vi "flatten parameters.vi"(8 "Output Tag":string, 9 "Process Variable Tag":string, 10 "Setpoint Tag":string, 11 "ID":string) -> (3 "wrapped data":string)   [LabVIEW 2014, in "PID Loop.lvclass"]
uses:
  PID Loop.lvclass
  String Parameters.ctl
  <vilib>/NI/Configuration Framework/serializable configuration/NISE_CEF_serializable configuration.lvclass
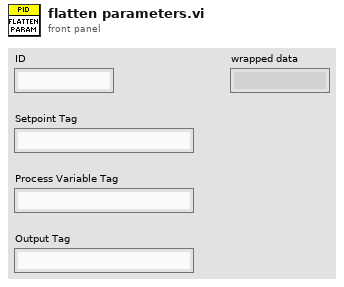
[diagram p1: front panel]
types:
  T1 = typedef "PID Loop.lvclass/String Parameters.ctl" = enum16{"Setpoint", "Process Variable", "Output", "Proportional Gain", "Integral Time", "Derivative Time", "Range High", "Range Low"}
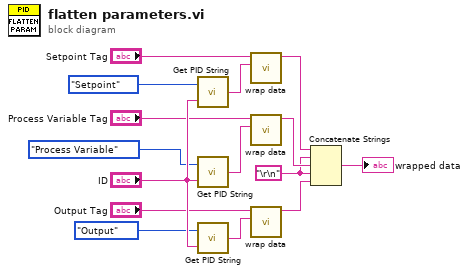
[diagram p0: block diagram]
diagram:
  w12 = "\r\n"
  n1 = call "Get PID String.vi"("PID Loop ID"="ID", "PID Parameter"=String_Parameters."Setpoint") -> ("Parameter String"=w5:string)
  n2 = call "Get PID String.vi"("PID Loop ID"="ID", "PID Parameter"=String_Parameters."Process Variable") -> ("Parameter String"=w6:string)
  n3 = call "Get PID String.vi"("PID Loop ID"="ID", "PID Parameter"=String_Parameters."Output") -> ("Parameter String"=w7:string)
  n4 = call <vilib>:"wrap data.vi"("identifier"=w5, "data to wrap"="Setpoint Tag") -> ("wrapped data"=w13:string)  [unwired: 9 in]
  n5 = call <vilib>:"wrap data.vi"("identifier"=w6, "data to wrap"="Process Variable Tag") -> ("wrapped data"=w14:string)  [unwired: 9 in]
  n6 = call <vilib>:"wrap data.vi"("identifier"=w7, "data to wrap"="Output Tag") -> ("wrapped data"=w15:string)  [unwired: 9 in]
  n7 = Concatenate Strings(w13, w12, w14, w12, w15) -> (→"wrapped data":string)
